vi "Max.vi"(6 "Search Lines":T2[](array[typedef]) {"Edge Info"."Distance (Real-World)" format="%.2f"; "Edge Info"."Location (Real-World)"."Y" format="%.2g"; "Edge Info"."Location (Real-World)"."X" format="%.2f"; "Edge Info"."Noise" format="%.2f"; "Edge Info"."Location (Pixel)"."Y" format="%.2g"; "Edge Info"."Location (Pixel)"."X" format="%.2f"; "Edge Info"."Strength" format="%.2f"; "Edge Info"."Distance (Pixel)" format="%.2f"}, 9 "Last Edges":T1[](array[typedef]) {"Distance (Real-World)" format="%.2f"; "Location (Real-World)"."Y" format="%.2g"; "Location (Real-World)"."X" format="%.2f"; "Noise" format="%.2f"; "Location (Pixel)"."Y" format="%.2g"; "Location (Pixel)"."X" format="%.2f"; "Strength" format="%.2f"; "Distance (Pixel)" format="%.2f"}, 10 "First Edges":T1[](array[typedef]) {"Distance (Real-World)" format="%.2f"; "Location (Real-World)"."Y" format="%.2g"; "Location (Real-World)"."X" format="%.2f"; "Noise" format="%.2f"; "Location (Pixel)"."Y" format="%.2g"; "Location (Pixel)"."X" format="%.2f"; "Strength" format="%.2f"; "Distance (Pixel)" format="%.2f"}, 11 "Refnum in":T3) -> (2 "Array":cluster{"X":sgl, "Y":sgl}[](array[cluster]), 3 "Numeric":sgl)   [LabVIEW 2014]
uses:
  <vilib>/vision/Image Controls.llb/IMAQ Image.ctl
  <vilib>/vision/Measure.llb/Search Line.ctl
  <vilib>/vision/Measure.llb/Edge New.ctl
  <vilib>/vision/NI_Vision_Development_Module.lvlib
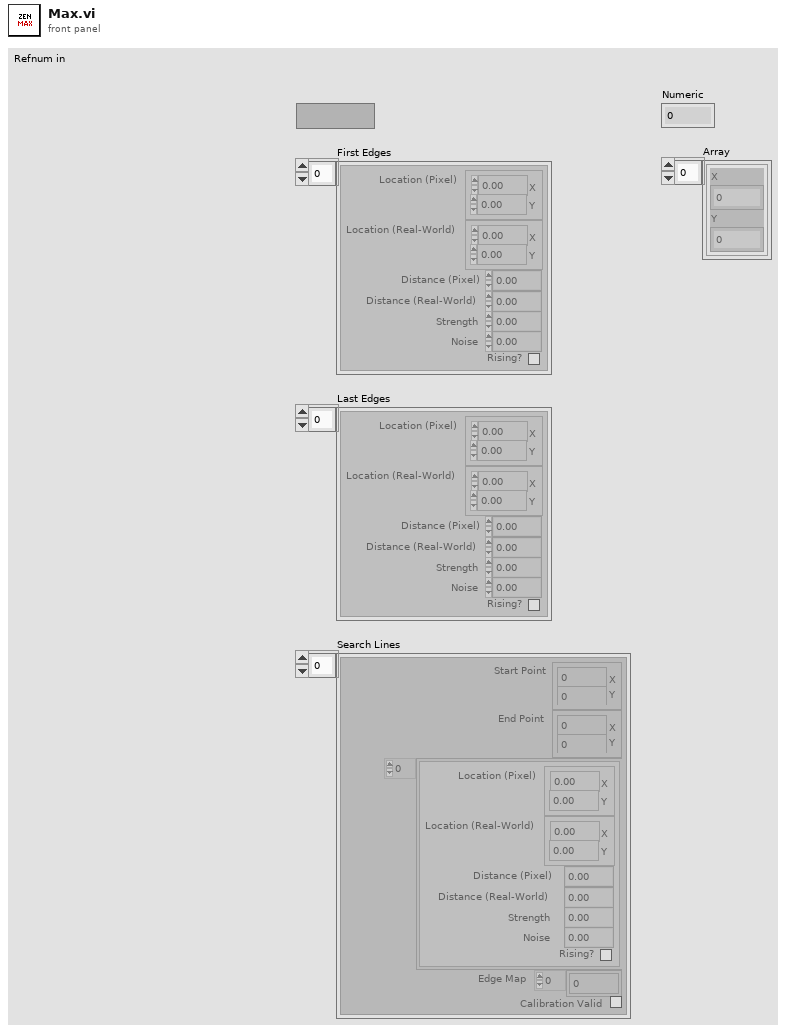
[diagram p1: front panel]
types:
  T1 = typedef "Edge New.ctl" = cluster{"Location (Pixel)":cluster{"X":sgl, "Y":sgl}, "Location (Real-World)":cluster{"X":sgl, "Y":sgl}, "Distance (Pixel)":dbl, "Distance (Real-World)":dbl, "Strength":dbl, "Noise":dbl, "Rising?":bool}
  T2 = typedef "Search Line.ctl" = cluster{"Start Point":cluster{"X":sgl, "Y":sgl}, "End Point":cluster{"X":sgl, "Y":sgl}, "Edge Info":T1[], "Edge Map":dbl[], "Calibration Valid":bool}
  T3 = typedef "IMAQ Image.ctl" = refnum<image>
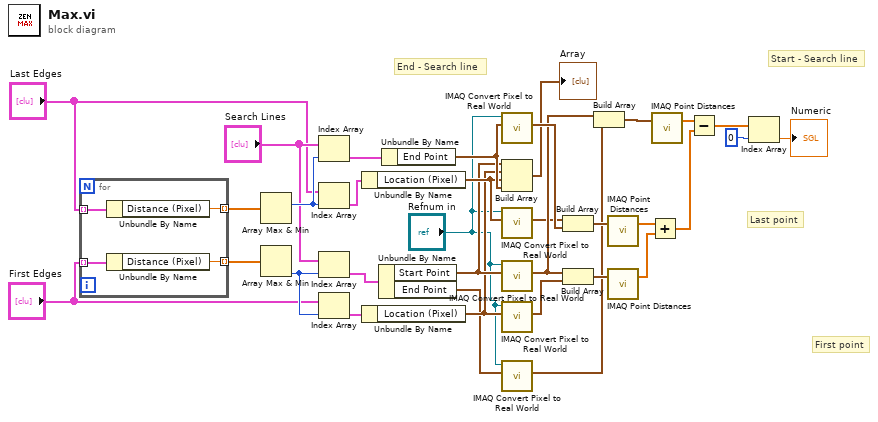
[diagram p0: block diagram]
diagram:
  # "Last point"
  # "First point"
  # "End - Search line"
  # "Start - Search line"
  n1 = for {
    tunnel: "First Edges" -> [w37] mode=indexing
    tunnel: [w36] -> w9 mode=indexing
    tunnel: "Last Edges" -> [w35] mode=indexing
    tunnel: [w34] -> w11 mode=indexing
    n2 = Unbundle By Name(w35) -> ("Distance (Pixel)"=w34:dbl)
    n3 = Unbundle By Name(w37) -> ("Distance (Pixel)"=w36:dbl)
  }
  n4 = Array Max & Min(array=w11) -> (max index (indices)=w15:i32)  [unwired: 3 out]
  n5 = Array Max & Min(array=w9) -> (min index (indices)=w12:i32)  [unwired: 3 out]
  n6 = Index Array(array="Search Lines", index=w15) -> (element=w14:T2)
  n7 = Index Array(array="Last Edges", index=w15) -> (element=w5:T1)
  n8 = Index Array(array="Search Lines", index=w12) -> (element=w6:T2)
  n9 = Index Array(array="First Edges", index=w12) -> (element=w4:T1)
  n10 = Unbundle By Name(w5) -> ("Location (Pixel)"=w20:cluster{"X":sgl, "Y":sgl})
  n11 = Unbundle By Name(w4) -> ("Location (Pixel)"=w16:cluster{"X":sgl, "Y":sgl})
  n12 = Unbundle By Name(w6) -> ("Start Point"=w17:cluster{"X":sgl, "Y":sgl}, "End Point"=w2:cluster{"X":sgl, "Y":sgl})
  n13 = Unbundle By Name(w14) -> ("End Point"=w21:cluster{"X":sgl, "Y":sgl})
  n14 = call "IMAQ Convert Pixel to Real World"("Pixel Coordinates"=w21, "Calibrated Image"="Refnum in") -> ("Real World Coordinates"=w29:cluster{"X":sgl, "Y":sgl})  [unwired: 4 in, 5 out]
  n15 = Build Array(w17, w16, w20, w21) -> (→"Array":cluster{"X":sgl, "Y":sgl}[])
  n16 = call "IMAQ Convert Pixel to Real World"("Pixel Coordinates"=w20, "Calibrated Image"="Refnum in") -> ("Real World Coordinates"=w22:cluster{"X":sgl, "Y":sgl})  [unwired: 4 in, 5 out]
  n17 = call "IMAQ Convert Pixel to Real World"("Pixel Coordinates"=w17, "Calibrated Image"="Refnum in") -> ("Real World Coordinates"=w28:cluster{"X":sgl, "Y":sgl})  [unwired: 4 in, 5 out]
  n18 = call "IMAQ Convert Pixel to Real World"("Pixel Coordinates"=w16, "Calibrated Image"="Refnum in") -> ("Real World Coordinates"=w18:cluster{"X":sgl, "Y":sgl})  [unwired: 4 in, 5 out]
  n19 = call "IMAQ Convert Pixel to Real World"("Pixel Coordinates"=w2, "Calibrated Image"="Refnum in") -> ("Real World Coordinates"=w1:cluster{"X":sgl, "Y":sgl})  [unwired: 4 in, 5 out]
  n20 = Build Array(w22, w29) -> (w23:cluster{"X":sgl, "Y":sgl}[])
  n21 = Build Array(w28, w18) -> (w19:cluster{"X":sgl, "Y":sgl}[])
  n22 = Build Array(w28, w1) -> (w30:cluster{"X":sgl, "Y":sgl}[])
  n23 = call "IMAQ Point Distances"("Points"=w23) -> ("Distances"=w24:sgl[])  [unwired: 4 in, 1 out]
  n24 = call "IMAQ Point Distances"("Points"=w19) -> ("Distances"=w25:sgl[])  [unwired: 4 in, 1 out]
  n25 = Add(x=w24, y=w25) -> (x+y=w26:sgl[])
  n26 = call "IMAQ Point Distances"("Points"=w30) -> ("Distances"=w31:sgl[])  [unwired: 4 in, 1 out]
  n27 = Subtract(x=w31, y=w26) -> (x-y=w27:sgl[])
  n28 = Index Array(array=w27, index=0) -> (element=→"Numeric":sgl)
